vi "myRIO_BRig_Host_TCP_parseCmd_getMessageType.vi"(9 "input_haveCmd":bool, 10 "input_countCmd":i32, 11 "input_strCmd":string) -> (3 "output_messageType":u8)   [LabVIEW 2014]
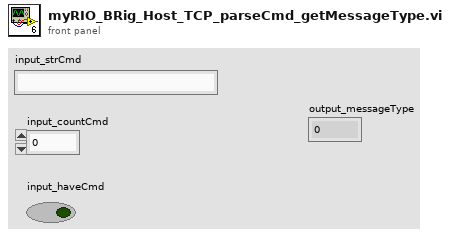
[diagram p1: front panel]
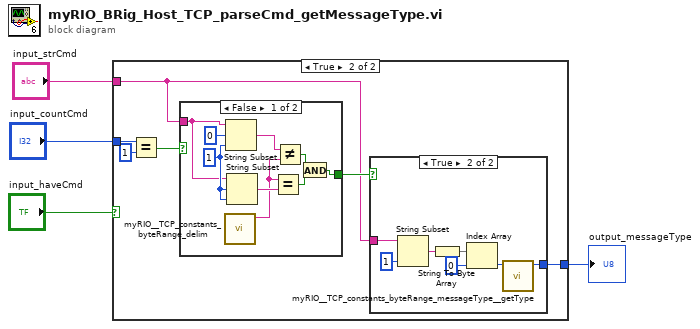
[diagram p0: block diagram]
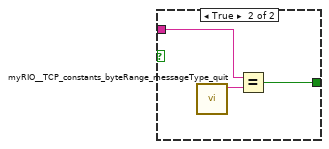
[diagram p3: hidden frame]
diagram:
  n1 = case shown="True" "input_haveCmd" {
    tunnel: "input_countCmd" -> [_ w8]
    tunnel: "input_strCmd" -> [_ w5]
    tunnel: [_ w9] -> w3
    frame False {
    }
    frame True {
      n2 = Equal?(x=w8, y=1) -> (x = y?=w6:bool)
      n3 = case shown="False" w6 {
        tunnel: [w19 w20] -> w10
        tunnel: w5 -> [w12 w21]
        frame False {
          w17 = 1 ("length (rest)")
          n4 = call "myRIO__TCP_constants_byteRange_delim.vi"() -> ("output_delim_char"=w11:string)  [unwired: 10 in, 1 out]
          n5 = String Subset(string=w12, offset (0)=0, length (rest)=w17) -> (substring=w15:string)
          n6 = String Subset(string=w12, offset (0)=w17, length (rest)=w17) -> (substring=w16:string)
          n7 = Equal?(x=w11, y=w16) -> (x = y?=w13:bool)
          n8 = Not Equal?(x=w15, y=w11) -> (x != y?=w14:bool)
          n9 = And(x=w14, y=w13) -> (x .and. y?=w19:bool)
        }
        frame True {
          n10 = call "myRIO__TCP_constants_byteRange_messageType_quit.vi"() -> ("output_Quit_char"=w22:string)  [unwired: 10 in, 1 out]
          n11 = Equal?(x=w21, y=w22) -> (x = y?=w20:bool)
        }
      }
      n12 = case shown="True" w10 {
        tunnel: [_ w24] -> w9
        tunnel: w5 -> [_ w23]
        frame False {
        }
        frame True {
          n13 = String Subset(string=w23, length (rest)=1 ("length (rest)")) -> (substring=w28:string)  [unwired: 1 in]
          n14 = String To Byte Array(string=w28) -> (unsigned byte array=w27:u8[])
          n15 = Index Array(array=w27, index=0) -> (element=w25:u8)
          n16 = call "myRIO__TCP_constants_byteRange_messageType__getType.vi"("input_byte"=w25) -> ("output_messageType"=w24:u8)  [unwired: 10 in]
        }
      }
    }
  }
  "output_messageType" <- w3
